vi "DataReceiver.vi"() -> ()   [LabVIEW 2010]
panel:
  in  "ClusDispQueue":refnum<queue>
  in  "ChanDispQueue":refnum<queue>
  in  "name (unnamed)":string
  in  "queue out":refnum<queue>
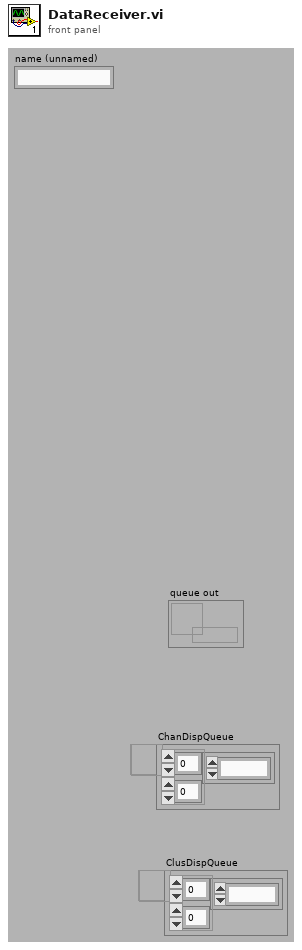
[diagram p1: front panel]
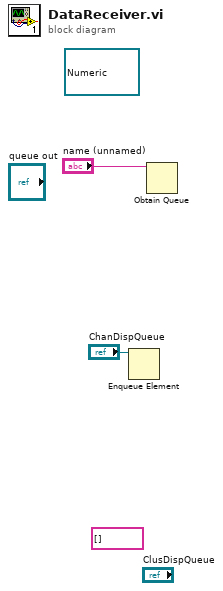
[diagram p0: block diagram]
diagram:
  (unwired) refnum<queue> refnum ("Network Queue")
  (unwired) string[] []
  n1 = Enqueue Element(queue="ChanDispQueue") -> ()  [unwired: 3 in, 3 out]
  n2 = Obtain Queue(name (unnamed)="name (unnamed)") -> ()  [unwired: 4 in, 3 out]
